vi "Filter Versions.vi"(8 "error in (no error)":errorcluster, 10 "Version Range":string, 11 "Semvers in":refnum<class "Semver.lvclass">[](array[class])) -> (0 "error out":errorcluster, 2 "Pointers":i32[](array[numeric]), 3 "Filtered Semvers":refnum<class "Semver.lvclass">[](array[class]))   [LabVIEW 2017, in "Semver.lvlib" / "Semver.lvclass"]
uses:
  Semver.lvclass
  Semver.lvclass/Semver.ctl
  Parse Number.vi
  <vilib>/Utility/error.llb/Error Cluster From Error Code.vi
  <vilib>/ErrorRing/Error Ring.xnode
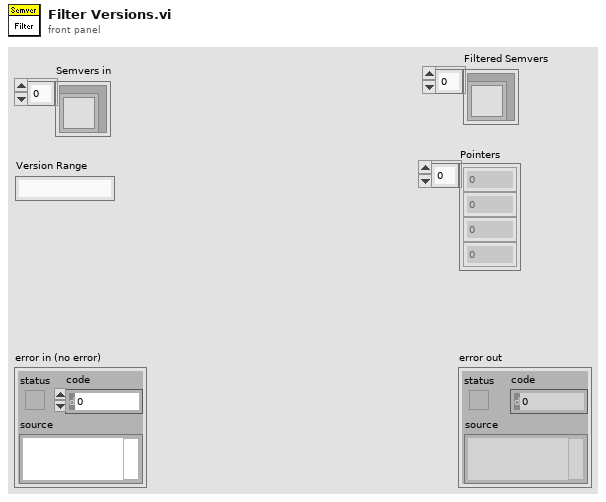
[diagram p1: front panel]
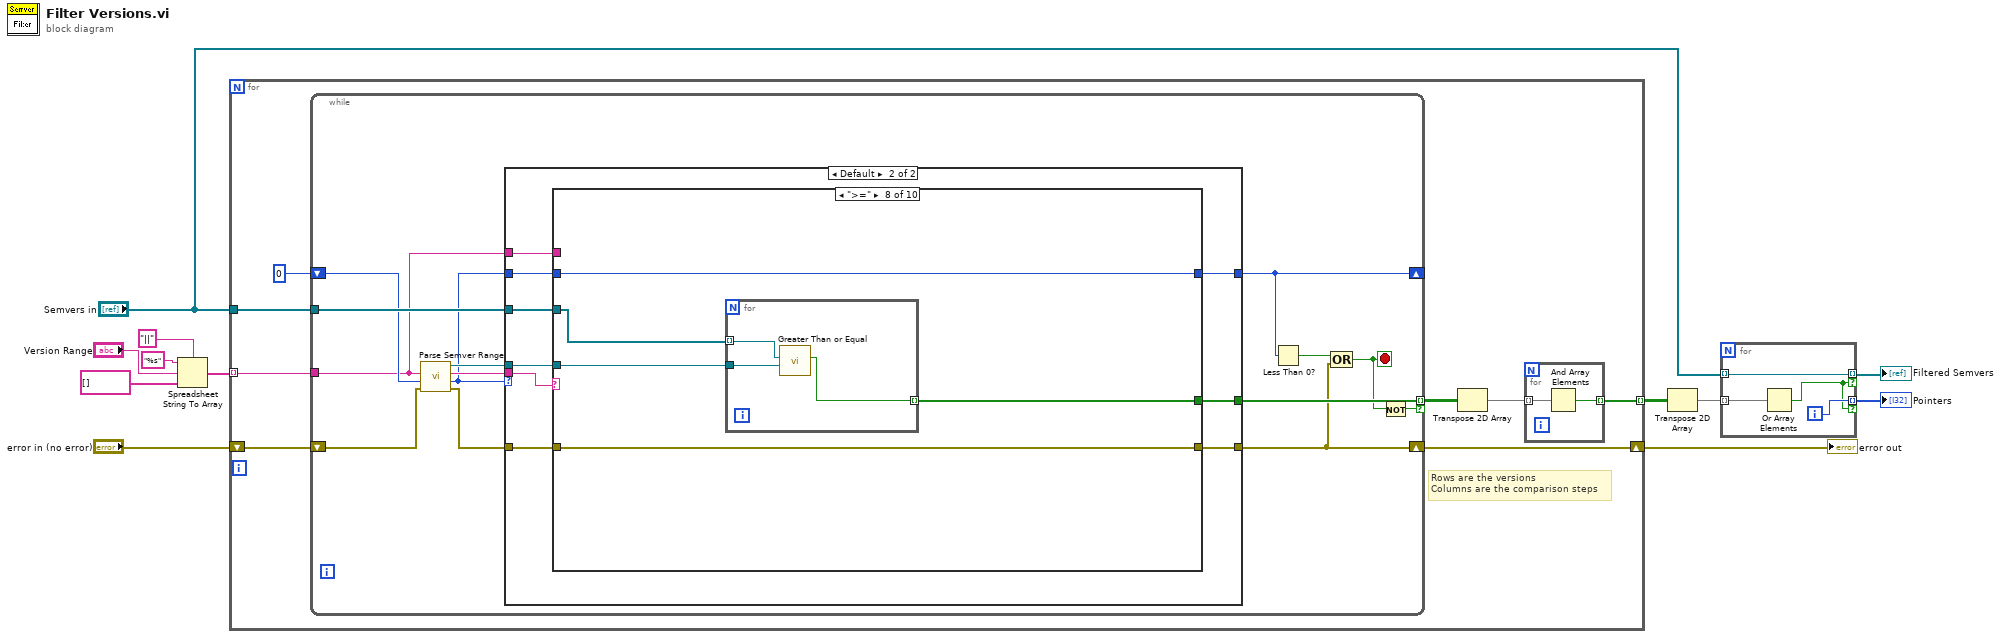
[diagram p0: block diagram]
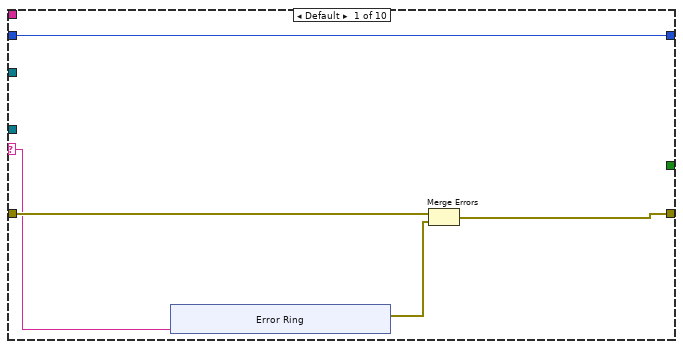
[diagram p3: hidden frame]
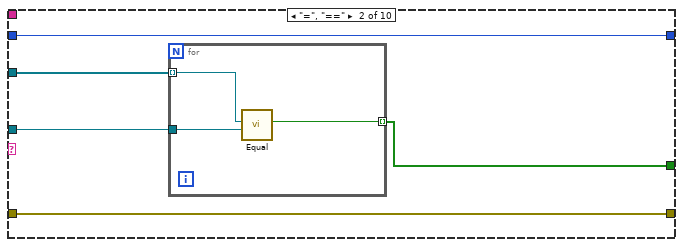
[diagram p4: hidden frame]
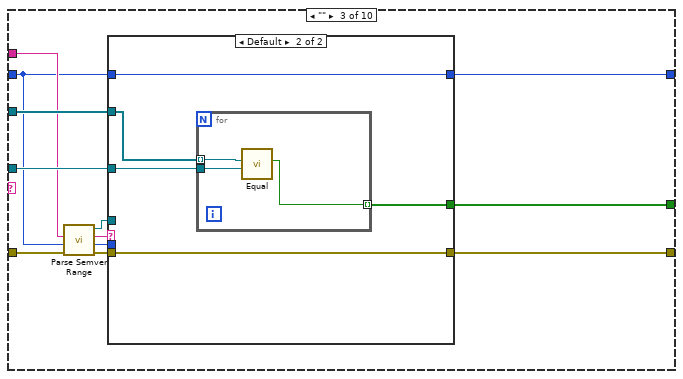
[diagram p5: hidden frame]
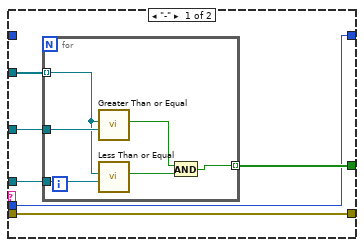
[diagram p6: hidden frame]
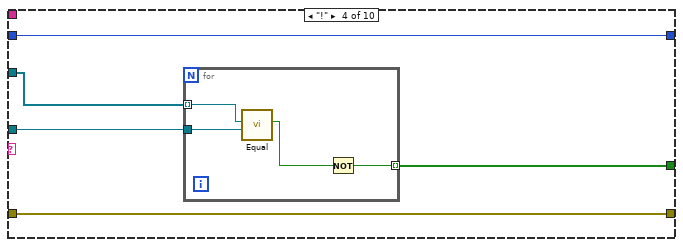
[diagram p7: hidden frame]
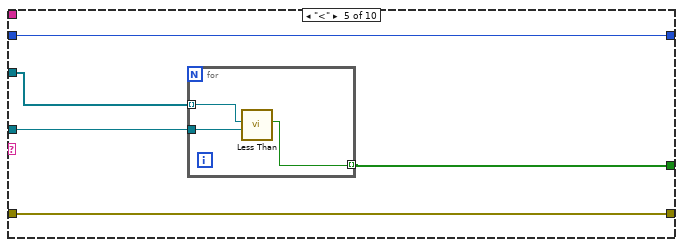
[diagram p8: hidden frame]
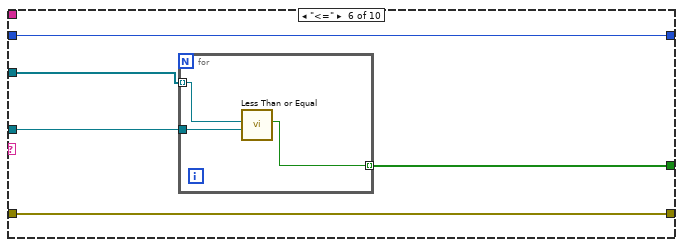
[diagram p9: hidden frame]
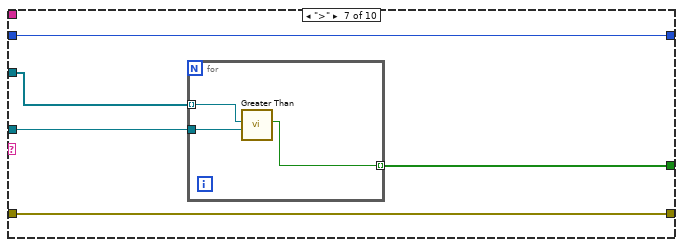
[diagram p10: hidden frame]
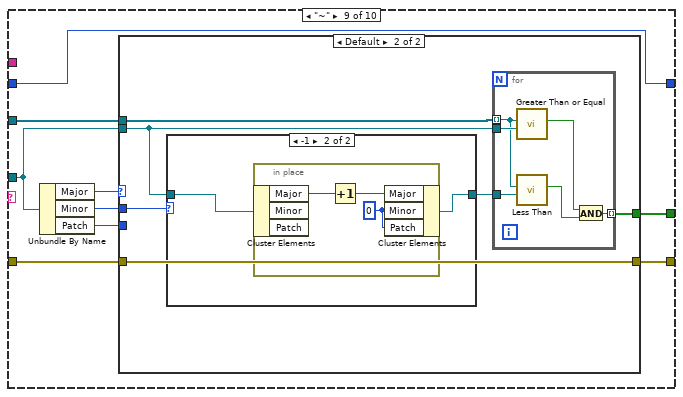
[diagram p11: hidden frame]
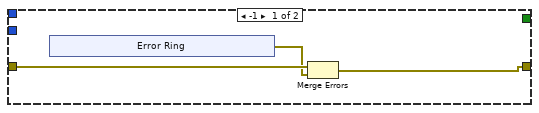
[diagram p12: hidden frame]
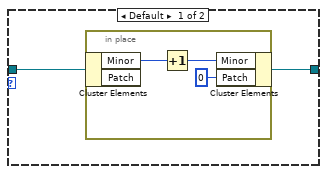
[diagram p13: hidden frame]
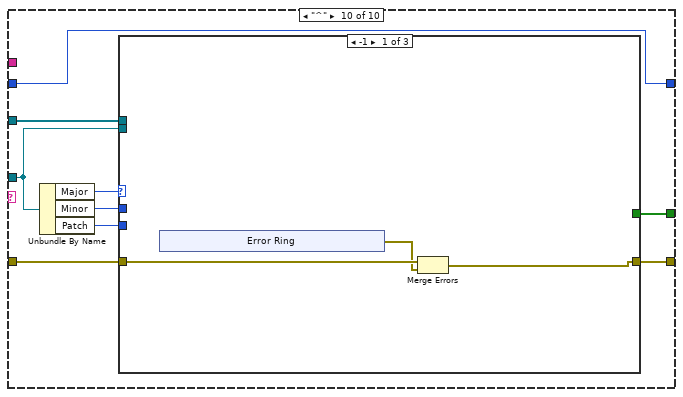
[diagram p14: hidden frame]
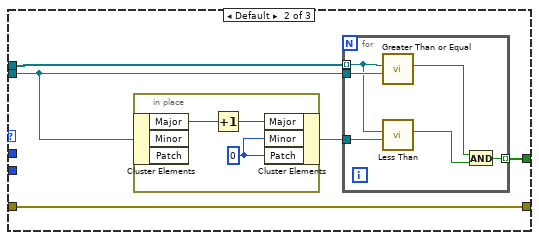
[diagram p15: hidden frame]
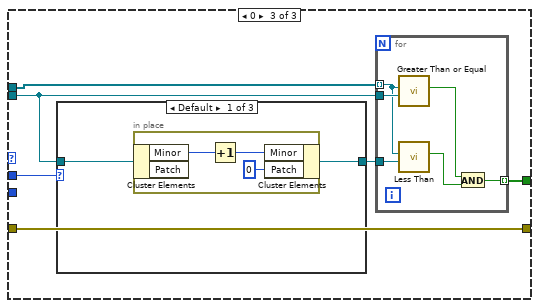
[diagram p16: hidden frame]
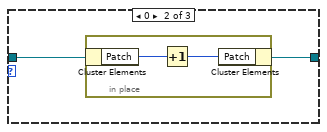
[diagram p17: hidden frame]
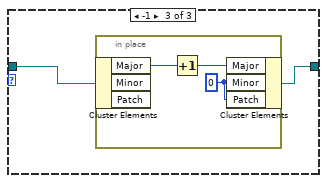
[diagram p18: hidden frame]
diagram:
  n1 = Spreadsheet String To Array(delimiter (Tab)="||", format string="%s", spreadsheet string="Version Range", array type (2D Dbl)=string[] []) -> (array=w6:string[])
  n2 = for {
    shift-right: [w18] -> w11
    shift-left: "error in (no error)" -> [w17]
    tunnel: w6 -> [w19] mode=indexing
    tunnel: "Semvers in" -> [w20]
    tunnel: [w13] -> w5 mode=indexing
    # "Rows are the versions\nColumns are the comparison steps"
    n3 = while {
      tunnel: [w29] -> w15 mode=indexing if=w23
      tunnel: w19 -> [w28]
      shift-right: [w25] -> w18
      shift-left: w17 -> [w33]
      shift-right: [w26] -> _
      shift-left: 0 ("Offset out") -> [w31]
      tunnel: w20 -> [w36]
      stop <- w24 stop-if-true
      n4 = call "Parse Semver Range.vi"("error in (no error)"=w33, "Offset in"=w31, "Range Specifier"=w28) -> ("error out"=w32:errorcluster, "Offset out"=w27:i32, "Operator"=w34:string, "Semver out"=w35:refnum<class "Semver.lvclass">)  [unwired: 5 in]
      n5 = case shown="Default" w27 {
        tunnel: w36 -> [_ w47]
        tunnel: [_ w46] -> w29
        tunnel: w35 -> [_ w45]
        tunnel: w34 -> [_ w44]
        tunnel: [w38 w43] -> w25
        tunnel: w32 -> [w38 w42]
        tunnel: w28 -> [_ w41]
        tunnel: w27 -> [w37 w40]
        tunnel: [w37 w39] -> w26
        frame -1 {
        }
        frame Default {
          n6 = case shown="\">=\"" w44 {
            selector: w44 -> [w51 _ _ _ _ _ _ _ _ _]
            tunnel: w47 -> [_ w64 w79 w100 w110 w118 w126 w134 w148 w187]
            tunnel: [_ w60 w68 w101 w109 w117 w125 w133 w141 w180] -> w46
            tunnel: w45 -> [_ w63 w78 w104 w113 w121 w129 w137 w149 w188]
            tunnel: [w50 w62 w75 w103 w112 w120 w128 w136 w146 w185] -> w43
            tunnel: w42 -> [w52 w62 w77 w103 w112 w120 w128 w136 w147 w186]
            tunnel: w41 -> [_ _ w76 _ _ _ _ _ _ _]
            tunnel: w40 -> [w48 w61 w70 w102 w111 w119 w127 w135 w142 w181]
            tunnel: [w48 w61 w71 w102 w111 w119 w127 w135 w142 w181] -> w39
            frame Default {
              n7 = xnode "Error Ring"("parameter 0"=w51) -> ("error out"=w49:errorcluster)
              n8 = Merge Errors(w52, w49) -> (w50:errorcluster)
            }
            frame "=", "==" {
              n9 = for {
                tunnel: w64 -> [w66] mode=indexing
                tunnel: w63 -> [w67]
                tunnel: [w65] -> w60 mode=indexing
                n10 = call "Equal.vi"("Semver 2"=w67, "Semver 1"=w66) -> ("Version 1 = Version 2"=w65:bool)  [unwired: 9 in]
              }
            }
            frame "" {
              n11 = call "Parse Semver Range.vi"("error in (no error)"=w77, "Offset in"=w70, "Range Specifier"=w76) -> ("error out"=w74:errorcluster, "Offset out"=w69:i32, "Operator"=w73:string, "Semver out"=w72:refnum<class "Semver.lvclass">)  [unwired: 5 in]
              n12 = case shown="Default" w73 {
                tunnel: w79 -> [w80 w92]
                tunnel: w78 -> [w85 w96]
                tunnel: [w82 w95] -> w68
                tunnel: [w84 w94] -> w75
                tunnel: w74 -> [w84 w94]
                tunnel: w72 -> [w83 _]
                tunnel: [w81 w93] -> w71
                tunnel: w70 -> [_ w93]
                tunnel: w69 -> [w81 _]
                frame "-" {
                  n13 = for {
                    tunnel: w85 -> [w91]
                    tunnel: w83 -> [w90]
                    tunnel: [w87] -> w82 mode=indexing
                    tunnel: w80 -> [w86] mode=indexing
                    n14 = call "Greater Than or Equal.vi"("Semver 2"=w91, "Semver 1"=w86) -> ("Version 1 >= Version 2"=w88:bool)  [unwired: 9 in]
                    n15 = call "Less Than or Equal.vi"("Semver 2"=w90, "Semver 1"=w86) -> ("Version 1 <= Version 2"=w89:bool)  [unwired: 9 in]
                    n16 = And(x=w88, y=w89) -> (x .and. y?=w87:bool)
                  }
                }
                frame Default {
                  n17 = for {
                    tunnel: w96 -> [w99]
                    tunnel: [w98] -> w95 mode=indexing
                    tunnel: w92 -> [w97] mode=indexing
                    n18 = call "Equal.vi"("Semver 2"=w99, "Semver 1"=w97) -> ("Version 1 = Version 2"=w98:bool)  [unwired: 9 in]
                  }
                }
              }
            }
            frame "!" {
              n19 = for {
                tunnel: w104 -> [w108]
                tunnel: [w106] -> w101 mode=indexing
                tunnel: w100 -> [w105] mode=indexing
                n20 = call "Equal.vi"("Semver 2"=w108, "Semver 1"=w105) -> ("Version 1 = Version 2"=w107:bool)  [unwired: 9 in]
                n21 = Not(x=w107) -> (.not. x?=w106:bool)
              }
            }
            frame "<" {
              n22 = for {
                tunnel: w113 -> [w116]
                tunnel: w110 -> [w115] mode=indexing
                tunnel: [w114] -> w109 mode=indexing
                n23 = call "Less Than.vi"("Semver 2"=w116, "Semver 1"=w115) -> ("Version 1 < Version 2"=w114:bool)  [unwired: 9 in]
              }
            }
            frame "<=" {
              n24 = for {
                tunnel: w121 -> [w124]
                tunnel: w118 -> [w123] mode=indexing
                tunnel: [w122] -> w117 mode=indexing
                n25 = call "Less Than or Equal.vi"("Semver 2"=w124, "Semver 1"=w123) -> ("Version 1 <= Version 2"=w122:bool)  [unwired: 9 in]
              }
            }
            frame ">" {
              n26 = for {
                tunnel: w129 -> [w132]
                tunnel: w126 -> [w131] mode=indexing
                tunnel: [w130] -> w125 mode=indexing
                n27 = call "Greater Than.vi"("Semver 2"=w132, "Semver 1"=w131) -> ("Version 1 > Version 2"=w130:bool)  [unwired: 9 in]
              }
            }
            frame ">=" {
              n28 = for {
                tunnel: w137 -> [w140]
                tunnel: w134 -> [w139] mode=indexing
                tunnel: [w138] -> w133 mode=indexing
                n29 = call "Greater Than or Equal.vi"("Semver 2"=w140, "Semver 1"=w139) -> ("Version 1 >= Version 2"=w138:bool)  [unwired: 9 in]
              }
            }
            frame "~" {
              n30 = Unbundle By Name(w149) -> ("Major"=w145:i32, "Minor"=w144:i32, "Patch"=w143:i32)
              n31 = case shown="Default" w145 {
                tunnel: w149 -> [_ w159]
                tunnel: [_ w163] -> w141
                tunnel: w148 -> [_ w158]
                tunnel: w147 -> [w152 w162]
                tunnel: [w151 w162] -> w146
                tunnel: w144 -> [_ w161]
                tunnel: w143 -> [_ _]
                frame -1 {
                  n32 = xnode "Error Ring"() -> ("error out"=w150:errorcluster)
                  n33 = Merge Errors(w152, w150) -> (w151:errorcluster)
                }
                frame Default {
                  n34 = case shown="-1" w161 {
                    tunnel: [w170 w175] -> w160
                    tunnel: w159 -> [w171 w176]
                    frame Default {
                      n35 = in-place {
                        n36 = in-place-cluster #1(w171) -> ("Minor"=w174:i32)  [unwired: 1 out]
                        n37 = Increment(x=w174) -> (x+1=w173:i32)
                        n38 = in-place-cluster #1("Minor"=w173, "Patch"=0) -> (w170:refnum<class "Semver.lvclass">)
                      }
                    }
                    frame -1 {
                      n39 = in-place {
                        w177 = 0 ("Minor")
                        n40 = in-place-cluster #2(w176) -> ("Major"=w179:i32)  [unwired: 2 out]
                        n41 = Increment(x=w179) -> (x+1=w178:i32)
                        n42 = in-place-cluster #2("Major"=w178, "Minor"=w177, "Patch"=w177) -> (w175:refnum<class "Semver.lvclass">)
                      }
                    }
                  }
                  n43 = for {
                    tunnel: [w169] -> w163 mode=indexing
                    tunnel: w160 -> [w166]
                    tunnel: w159 -> [w165]
                    tunnel: w158 -> [w164] mode=indexing
                    n44 = call "Greater Than or Equal.vi"("Semver 2"=w165, "Semver 1"=w164) -> ("Version 1 >= Version 2"=w168:bool)  [unwired: 9 in]
                    n45 = call "Less Than.vi"("Semver 2"=w166, "Semver 1"=w164) -> ("Version 1 < Version 2"=w167:bool)  [unwired: 9 in]
                    n46 = And(x=w168, y=w167) -> (x .and. y?=w169:bool)
                  }
                }
              }
            }
            frame "^" {
              n47 = Unbundle By Name(w188) -> ("Major"=w184:i32, "Minor"=w183:i32, "Patch"=w182:i32)
              n48 = case shown="-1" w184 {
                tunnel: w188 -> [_ w198 w212]
                tunnel: [_ w201 w216] -> w180
                tunnel: w187 -> [_ w197 w211]
                tunnel: w186 -> [w191 w200 w215]
                tunnel: [w190 w200 w215] -> w185
                tunnel: w183 -> [_ _ w214]
                tunnel: w182 -> [_ _ _]
                frame -1 {
                  n49 = xnode "Error Ring"() -> ("error out"=w189:errorcluster)
                  n50 = Merge Errors(w191, w189) -> (w190:errorcluster)
                }
                frame Default {
                  n51 = in-place {
                    w208 = 0 ("Patch")
                    n52 = in-place-cluster #3(w198) -> ("Major"=w210:i32)  [unwired: 2 out]
                    n53 = Increment(x=w210) -> (x+1=w209:i32)
                    n54 = in-place-cluster #3("Major"=w209, "Minor"=w208, "Patch"=w208) -> (w199:refnum<class "Semver.lvclass">)
                  }
                  n55 = for {
                    tunnel: [w207] -> w201 mode=indexing
                    tunnel: w199 -> [w204]
                    tunnel: w198 -> [w203]
                    tunnel: w197 -> [w202] mode=indexing
                    n56 = call "Greater Than or Equal.vi"("Semver 2"=w203, "Semver 1"=w202) -> ("Version 1 >= Version 2"=w206:bool)  [unwired: 9 in]
                    n57 = call "Less Than.vi"("Semver 2"=w204, "Semver 1"=w202) -> ("Version 1 < Version 2"=w205:bool)  [unwired: 9 in]
                    n58 = And(x=w206, y=w205) -> (x .and. y?=w207:bool)
                  }
                }
                frame 0 {
                  n59 = case shown="Default" w214 {
                    tunnel: [w223 w228 w232] -> w213
                    tunnel: w212 -> [w224 w229 w233]
                    frame Default {
                      n60 = in-place {
                        n61 = in-place-cluster #4(w224) -> ("Minor"=w227:i32)  [unwired: 1 out]
                        n62 = Increment(x=w227) -> (x+1=w226:i32)
                        n63 = in-place-cluster #4("Minor"=w226, "Patch"=0) -> (w223:refnum<class "Semver.lvclass">)
                      }
                    }
                    frame 0 {
                      n64 = in-place {
                        n65 = in-place-cluster #5(w229) -> ("Patch"=w231:i32)
                        n66 = Increment(x=w231) -> (x+1=w230:i32)
                        n67 = in-place-cluster #5("Patch"=w230) -> (w228:refnum<class "Semver.lvclass">)
                      }
                    }
                    frame -1 {
                      n68 = in-place {
                        w234 = 0 ("Minor")
                        n69 = in-place-cluster #6(w233) -> ("Major"=w236:i32)  [unwired: 2 out]
                        n70 = Increment(x=w236) -> (x+1=w235:i32)
                        n71 = in-place-cluster #6("Major"=w235, "Minor"=w234, "Patch"=w234) -> (w232:refnum<class "Semver.lvclass">)
                      }
                    }
                  }
                  n72 = for {
                    tunnel: [w222] -> w216 mode=indexing
                    tunnel: w213 -> [w219]
                    tunnel: w212 -> [w218]
                    tunnel: w211 -> [w217] mode=indexing
                    n73 = call "Greater Than or Equal.vi"("Semver 2"=w218, "Semver 1"=w217) -> ("Version 1 >= Version 2"=w221:bool)  [unwired: 9 in]
                    n74 = call "Less Than.vi"("Semver 2"=w219, "Semver 1"=w217) -> ("Version 1 < Version 2"=w220:bool)  [unwired: 9 in]
                    n75 = And(x=w221, y=w220) -> (x .and. y?=w222:bool)
                  }
                }
              }
            }
          }
        }
      }
      n76 = Less Than 0?(x=w26) -> (x < 0?=w30:bool)
      n77 = Compound Arithmetic op=OR(w30, w25) -> (w24:bool)
      n78 = Not(x=w24) -> (.not. x?=w23:bool)
    }
    n79 = Transpose 2D Array(2D array=w15) -> (transposed array=w14:bool[][])
    n80 = for {
      tunnel: w14 -> [w22] mode=indexing
      tunnel: [w21] -> w13 mode=indexing
      n81 = And Array Elements(Boolean array=w22) -> (logical AND=w21:bool)
    }
  }
  "error out" <- w11
  n82 = Transpose 2D Array(2D array=w5) -> (transposed array=w4:bool[][])
  n83 = for {
    tunnel: w4 -> [w239] mode=indexing
    tunnel: "Semvers in" -> [w240] mode=indexing
    tunnel: [w240] -> w2 mode=indexing if=w237
    tunnel: [w238] -> w1 mode=indexing if=w237
    i -> [w238]
    n84 = Or Array Elements(Boolean array=w239) -> (logical OR=w237:bool)
  }
  "Filtered Semvers" <- w2
  "Pointers" <- w1
